vi "Configure Signal (with char data).vi"(0 "Register Bus":T4, 1 "scope":string(combo)="rx", 2 "Characterization Data":T1 {"Frequencies [Hz]" format="%#_6p"}, 5 "sample rate [S/s]":dbl=10000000.0 caption="Sample Rate [S/s]" min=1.0 max=250000000.0 format="%#.3pS/s", 7 "frequency [Hz]":dbl=2450000000.0 caption="Frequency [Hz]" format="%#.3pHz", 9 "level [dBm]":dbl=-10.0 caption="Level [dBm]" format="%#_gdBm", 11 "error in":errorcluster, 12 "LO source":string(combo)="LO1" caption="LO Source", 13 "LO frequency [Hz]":dbl=-1.0 caption="LO Frequency [Hz]" format="%#.3pHz") -> (3 "coerced vertical range [Vpp]":dbl caption="Coerced Vertical Range [Vpp]" format="%#.3pV", 4 "Register Bus (out)":T4, 6 "coerced sample rate [S/s]":dbl=10000000.0 caption="Coerced Sample Rate [S/s]" min=1.0 max=250000000.0 format="%#.3pS/s", 8 "coerced frequency [Hz]":dbl=2450000000.0 caption="Coerced Frequency [Hz]" format="%#.3pHz", 10 "coerced level [dBm]":dbl=-10.0 caption="Coerced Level [dBm]" format="%#_gdBm", 14 "coerced LO frequency [Hz]":dbl=-1.0 caption="coerced LO Frequency [Hz]" format="%#.3pHz", 15 "error out":errorcluster)   [LabVIEW 2017]
doc: "Configure the DSP and signal path for the device with characterization data."
uses:
  <instrlib>/_niInstr/Register Bus/v0/Host/Public/Register Bus Session.ctl
  <instrlib>/_niInstr/Register Bus/v0/Host/Private/Session Data.ctl
  <instrlib>/ni579x/Config/v2/Shared/Types/ni579x Characterization Data.ctl
  <instrlib>/ni579x/Config/v2/Shared/Types/ni579x IQ Imbalance.ctl
  <instrlib>/ni579x/Config/v2/Shared/Types/ni579x Gain to Attenuation Mapping.ctl
  Rx FPGA VI Reference.ctl
  Tx FPGA VI Reference.ctl
  <vilib>/Utility/error.llb/Error Cluster From Error Code.vi
  <vilib>/rvi/errors/niLvFpgaAdjustHostInterfaceError.vi
  <vilib>/rvi/interface/nirviReadWriteControl/nirviReadWriteControl.xnode
  <instrlib>/ni579x/Config/v2/Host/ni579x Config v2 Host.lvlib
  NiFpgaLv.dll
  <vilib>/rvi/interface/Simulation/niFpgaSimulationCallBeginRW.vi
  <instrlib>/_niInstr/Register Bus/v0/Host/niInstr Register Bus v0 Host.lvlib
  <instrlib>/ni579x/Config/v2/Shared/ni579x Config v2 Shared.lvlib
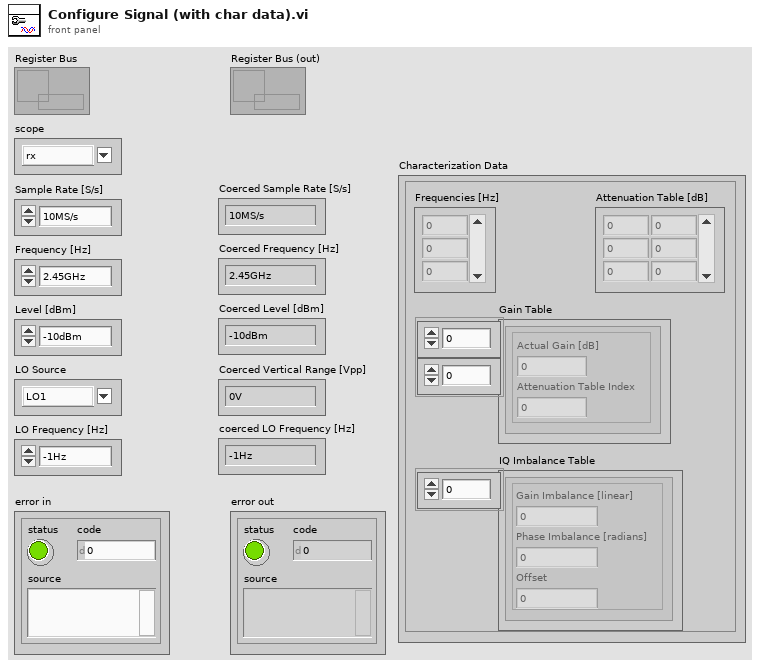
[diagram p1: front panel]
types:
  T1 = typedef "ni579x Config v2 Shared.lvlib/ni579x Characterization Data.ctl" = cluster{"Attenuation Table [dB]":dbl[][], "Frequencies [Hz]":dbl[], "IQ Imbalance Table":T2[], "Gain Table":T3[][]}
  T2 = typedef "ni579x Config v2 Shared.lvlib/ni579x IQ Imbalance.ctl" = cluster{"Gain Imbalance [linear]":dbl, "Phase Imbalance [radians]":dbl, "Offset":cdb}
  T3 = typedef "ni579x Config v2 Shared.lvlib/ni579x Gain to Attenuation Mapping.ctl" = cluster{"Actual Gain [dB]":dbl, "Attenuation Table Index":i32}
  T4 = typedef "niInstr Register Bus v0 Host.lvlib/Register Bus Session.ctl" = refnum<queue>
  T5 = typedef "niInstr DSP v1 Shared.lvlib/IQ Gain.ctl" = cluster{"gain I":fxp<+/-,24,3>, "gain Q":fxp<+/-,24,3>}
  T6 = typedef "niInstr DSP v1 Shared.lvlib/IQ Impairments.ctl" = cluster{"inline gain I":fxp<+/-,18,1>, "inline gain Q":fxp<+/-,18,1>, "cross gain I":fxp<+/-,18,1>, "cross gain Q":fxp<+/-,18,1>, "pre-gain offset I":fxp<+/-,18,1>, "pre-gain offset Q":fxp<+/-,18,1>, "post-gain offset I":fxp<+/-,18,1>, "post-gain offset Q":fxp<+/-,18,1>}
  T7 = typedef "Rx FPGA VI Reference.ctl" = refnum<k20>
  T8 = typedef "Tx FPGA VI Reference.ctl" = refnum<k20>
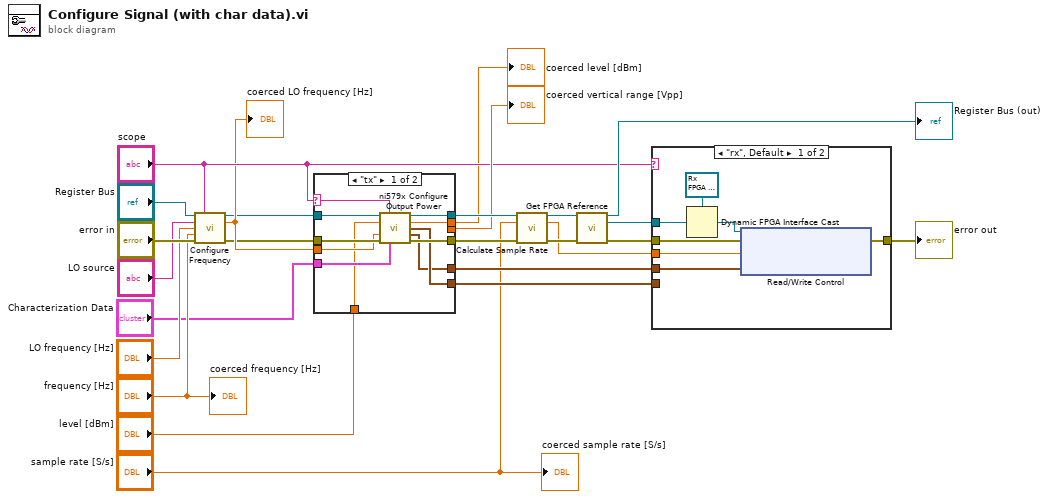
[diagram p0: block diagram]
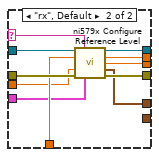
[diagram p2: hidden frame]
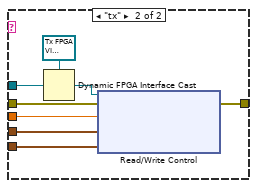
[diagram p3: hidden frame]
diagram:
  n1 = call "Configure Frequency.vi"("Register Bus"="Register Bus", "scope"="scope", "LO source"="LO source", "LO frequency [Hz]"="LO frequency [Hz]", "frequency [Hz]"="frequency [Hz]", "error in"="error in") -> ("Register Bus (out)"=w2:T4, "coerced LO frequency [Hz]"=w4:dbl, "error out"=w1:errorcluster)  [unwired: 7 in]
  "coerced LO frequency [Hz]" <- w4
  n2 = case shown="\"tx\"" "scope" {
    selector: "scope" -> [w30 w38]
    tunnel: w1 -> [w36 w47]
    tunnel: "level [dBm]" -> [w29 w46]
    tunnel: w2 -> [w32 w45]
    tunnel: [w35 w44] -> w18
    tunnel: [w31 w43] -> w17
    tunnel: [_ w42] -> w15
    tunnel: [w27 w41] -> w14
    tunnel: "Characterization Data" -> [w34 w40]
    tunnel: w4 -> [w33 w39]
    tunnel: [w28 _] -> w8
    tunnel: [w26 w37] -> w7
    frame "tx" {
      n3 = call <instrlib>:"ni579x Configure Output Power.vi"("Register Bus"=w32, "scope"=w30, "output power [dBm]"=w29, "frequency [Hz]"=w33, "Error In"=w36, "characterization data"=w34) -> ("Register Bus (out)"=w31:T4, "coerced output power [dBm]"=w26:dbl, "digital gain"=w28:T5, "IQ impairment correction"=w27:T6, "Error Out"=w35:errorcluster)  [unwired: 5 in]
    }
    frame "rx", Default {
      n4 = call <instrlib>:"ni579x Configure Reference Level.vi"("Register Bus"=w45, "scope"=w38, "reference level [dBm]"=w46, "frequency [Hz]"=w39, "Error In"=w47, "characterization data"=w40) -> ("Register Bus (out)"=w43:T4, "coerced reference level [dBm]"=w37:dbl, "coerced vertical range [Vpp]"=w42:dbl, "IQ impairment correction"=w41:T6, "Error Out"=w44:errorcluster)  [unwired: 5 in]
    }
  }
  "coerced vertical range [Vpp]" <- w15
  "coerced level [dBm]" <- w7
  n5 = call "Calculate Sample Rate.vi"("Register Bus"=w17, "sample rate [S/s]"="sample rate [S/s]", "error in"=w18) -> ("Register Bus (out)"=w19:T4, "sample rate [ratio]"=w24:dbl, "error out"=w25:errorcluster)  [unwired: 10 in]
  n6 = call <instrlib>:"Get FPGA Reference.vi"("session in"=w19, "error in"=w25) -> ("session out"=→"Register Bus (out)":T4, "fpga ref"=w23:refnum<k20>, "error out"=w21:errorcluster)  [unwired: 11 in]
  n7 = case shown="\"rx\", Default" "scope" {
    tunnel: w24 -> [w54 w62]
    tunnel: w23 -> [w53 w61]
    tunnel: [w52 w60] -> w22
    tunnel: w21 -> [w51 w59]
    tunnel: w14 -> [w48 w56]
    tunnel: w8 -> [_ w55]
    frame "rx", Default {
      n8 = Dynamic FPGA Interface Cast(Session In=T7 refnum ("FPGA VI Reference Out"), Type=w53) -> (Session Out=w49:T7)
      n9 = xnode "Read/Write Control"("FPGA VI Reference In"=w49, "error in"=w51, "rx.output sample rate"=w54, "rx.impairments"=w48) -> ("error out"=w52:errorcluster)  [unwired: 1 out]
    }
    frame "tx" {
      n10 = Dynamic FPGA Interface Cast(Session In=T8 refnum ("FPGA VI Reference Out"), Type=w61) -> (Session Out=w57:T8)
      n11 = xnode "Read/Write Control"("FPGA VI Reference In"=w57, "error in"=w59, "tx.input sample rate"=w62, "tx.impairments"=w56, "tx.gain"=w55) -> ("error out"=w60:errorcluster)  [unwired: 1 out]
    }
  }
  "error out" <- w22
  "coerced sample rate [S/s]" <- "sample rate [S/s]"
  "coerced frequency [Hz]" <- "frequency [Hz]"
